vi "zmq_getsocketopt_int.vi"(3 "error in":errorcluster, 4 "option":T1=enum."ZMQ_SWAP", 5 "socket in":refnum<class "zmq_socket.lvclass">) -> (0 "error out":errorcluster, 1 "value":i32, 2 "socket out":refnum<class "zmq_socket.lvclass">)   [LabVIEW 2010, in "zeromq.lvlib" / "zmq_socket.lvclass"]
doc: "Query the value of <b>option</b> for the given <b>socket</b>.\n\nYou are responsible for selecting the correct polymorphic instance for the option you wish to query. Most options return int32; check the API docs or code diagram.\n\nFurther API documentation: http://api.zeromq.org/3-2:zmq-getsockopt"
uses:
  zmq_socket.lvclass
  socket_options.ctl
  zmq_socket.lvclass/zmq_socket.ctl
  zeromq.lvlib
panel:
  # "ØMQ"
  # "labview"
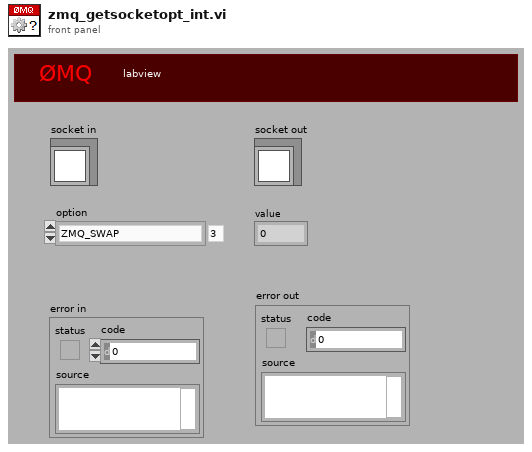
[diagram p1: front panel]
types:
  T1 = typedef "zeromq.lvlib/socket_options.ctl" = enum8{"NONE", "ZMQ_HWM", "<2>", "ZMQ_SWAP", "ZMQ_AFFINITY", "ZMQ_IDENTITY", "ZMQ_SUBSCRIBE", "ZMQ_UNSUBSCRIBE", "ZMQ_RATE", "ZMQ_RECOVERY_IVL", "ZMQ_MCAST_LOOP", "ZMQ_SNDBUF", "ZMQ_RCVBUF", "ZMQ_RCVMORE", "ZMQ_FD", "ZMQ_EVENTS", "ZMQ_TYPE", "ZMQ_LINGER", "ZMQ_RECONNECT_IVL", "ZMQ_BACKLOG", "ZMQ_RECOVERY_IVL_MSEC", "ZMQ_RECONNECT_IVL_MAX", "ZMQ_MAXMSGSIZE", "ZMQ_SNDHWM", "ZMQ_RCVHWM", "ZMQ_MULTICAST_HOPS", "<26>", "ZMQ_RCVTIMEO", "ZMQ_SNDTIMEO", "<29>", "<30>", "ZMQ_IPV4ONLY", "ZMQ_LAST_ENDPOINT", "ZMQ_ROUTER_MANDATORY", "ZMQ_TCP_KEEPALIVE", "ZMQ_TCP_KEEPALIVE_CNT", "ZMQ_TCP_KEEPALIVE_IDLE", "ZMQ_TCP_KEEPALIVE_INTVL", "ZMQ_TCP_ACCEPT_FILTER", "ZMQ_DELAY_ATTACH_ON_CONNECT", "ZMQ_XPUB_VERBOSE"}
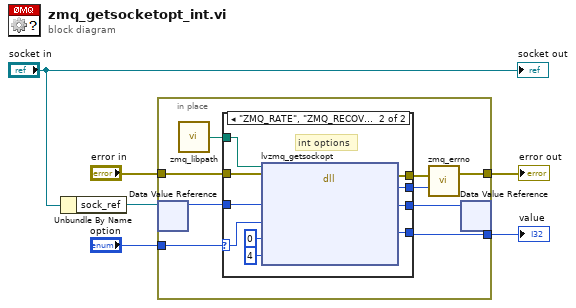
[diagram p0: block diagram]
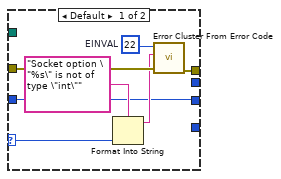
[diagram p2: hidden frame]
diagram:
  n1 = Unbundle By Name("socket in") -> ("sock_ref"=w1:refnum<data-value>)
  n2 = in-place {
    in-place-border: [w13] -> w6
    in-place-border: "error in" -> [w12]
    in-place-border: "option" -> [w11]
    in-place-border: [w10] -> w3
    n3 = in-place-dvr #1(w1) -> (w9:u64)  [unwired: 1 out]
    n4 = call "zmq_libpath.vi"() -> ("path"=w7:path)
    n5 = case shown="\"ZMQ_RATE\", \"ZMQ_RECOVERY_IVL\", \"ZMQ_SNDBUF\"..\"ZMQ_RECONNECT_IVL_MAX\", \"ZMQ_SNDHWM\"..\"ZMQ_MULTICAST_HOPS\", \"ZMQ_RCVTIMEO\", \"ZMQ_SNDTIMEO\", \"ZMQ_IPV4ONLY\", \"ZMQ_ROUTER_MANDATORY\"..\"ZMQ_XPUB_VERBOSE\"" w11 {
      selector: w11 -> [w19 w30]
      tunnel: [w22 w32] -> w15
      tunnel: [_ w31] -> w14
      tunnel: w12 -> [w20 w28]
      tunnel: [_ w26] -> w10
      tunnel: w9 -> [w16 w25]
      tunnel: [w16 w24] -> w8
      tunnel: w7 -> [_ w23]
      frame Default {
        w21 = 22  # EINVAL
        n6 = Format Into String(format string="Socket option \"%s\" is not of type \"int\"", w19) -> (resulting string=w17:string)  [unwired: 2 in, 1 out]
        n7 = call <vilib>:"Error Cluster From Error Code.vi"("error in (no error)"=w20, "error message (\"\")"=w17, "error code (0)"=w21) -> ("error out"=w22:errorcluster)  [unwired: 6 in]
      }
      frame "ZMQ_RATE", "ZMQ_RECOVERY_IVL", "ZMQ_SNDBUF".."ZMQ_RECONNECT_IVL_MAX", "ZMQ_SNDHWM".."ZMQ_MULTICAST_HOPS", "ZMQ_RCVTIMEO", "ZMQ_SNDTIMEO", "ZMQ_IPV4ONLY", "ZMQ_ROUTER_MANDATORY".."ZMQ_XPUB_VERBOSE" {
        # "int options"
        n8 = dll-call lib="?" fn="lvzmq_getsockopt"(path in=w23, error in=w28, "socket"=w25, "option"=w30, "data"=0, "len"=u32 4) -> (error out=w32:errorcluster, "return type"=w31:i32, "socket"=w24:u64, "data"=w26:i32)  [unwired: 3 in, 1 out]
      }
    }
    n9 = call "zmq_errno.vi"("retval"=w14, "error in"=w15) -> ("error out"=w13:errorcluster)  [unwired: 1 out]
    n10 = in-place-dvr #1(w8) -> ()  [unwired: 2 out]
  }
  "error out" <- w6
  "value" <- w3
  "socket out" <- "socket in"
